vi "Result_Test.vi"(8 "error in (no error)":errorcluster caption="entrée d'erreur (pas d'erreur)", 11 "Nodon_Get_Power IN":refnum<class "Nodon_Get_Power.lvclass">) -> (0 "error out":errorcluster caption="sortie d'erreur", 3 "Nodon_Get_Power OUT":refnum<class "Nodon_Get_Power.lvclass">)   [LabVIEW 2020, in "Library Test.lvlib" / "Nodon_Get_Power.lvclass"]
uses:
  Nodon_Get_Power.lvclass
  C:/Users/ngarcin/OneDrive - Altyor/Standard TB/Suite TB45/Class/Test/Test (Default)/Test (Default).lvclass
  Commun VI/TypeDef/Variable Printable.ctl
  JSON API/JSON Value/Set from JSON string.vi
  JSON API/JSON Value/JSON Value.lvclass
  Nodon_Send_Command_UART.lvclass
  JSON API/Variant JSON/Variant JSON.lvlib
  JSON API/Get Polymorphic/JSON GetSet.lvlib
  Commun VI/Library Commun.lvlib
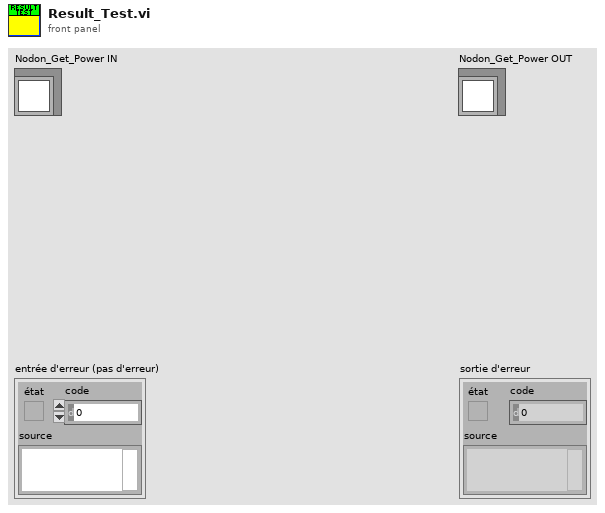
[diagram p1: front panel]
types:
  T1 = typedef "Variable Printable.ctl" = string
  T2 = enum16{"Get Variable", "Get All Variables", "Set Variable", "Delete Variable", "Delete All Variable"}
  T3 = cluster{"Commande Type":string, "Command ID":string, "Data":string, "Error":string}
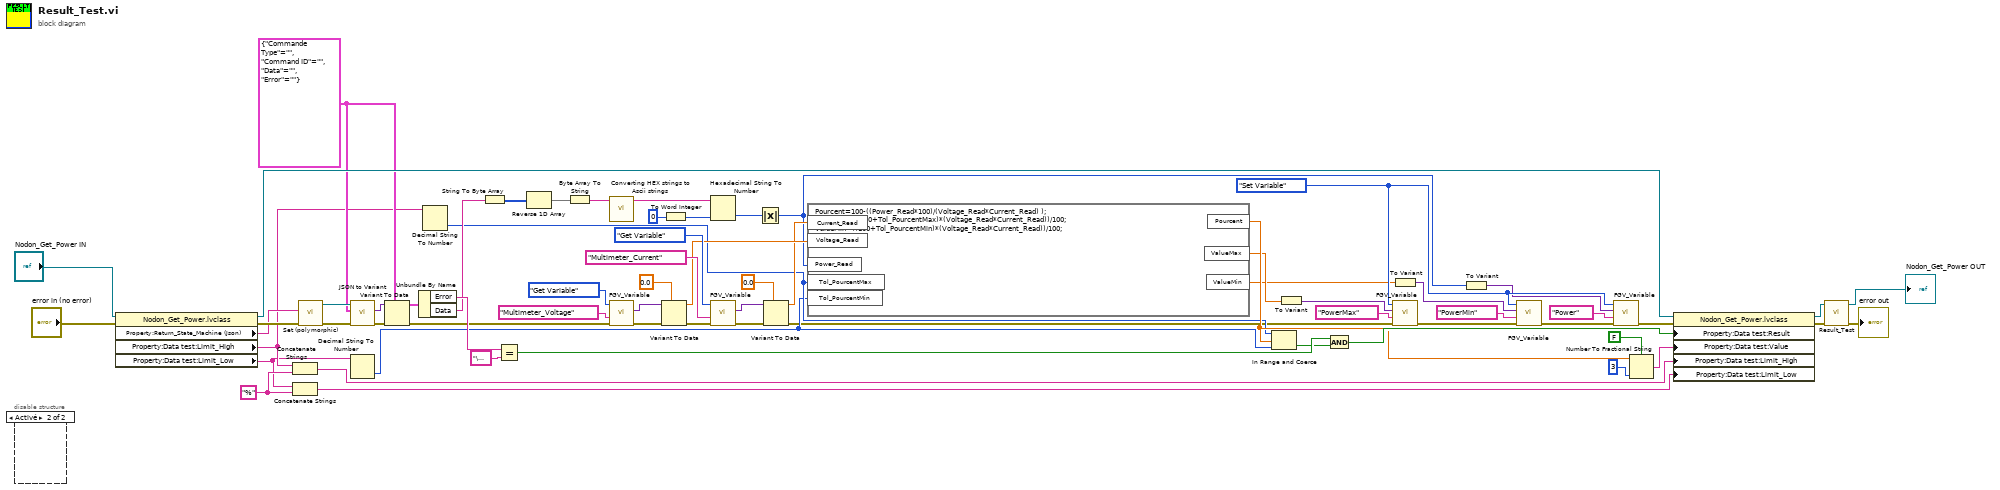
[diagram p0: block diagram]
diagram:
  w9 = T2."Set Variable" ("Function")
  w41 = "%" ("chaîne")
  w54 = T3 {"Commande Type"="", "Command ID"="", "Data"="", "Error"=""}
  n1 = disable-structure shown="Activé" {
    frame Disabled {
    }
    frame Enabled {
    }
  }
  n2 = property class="Nodon_Get_Power.lvclass"(reference="Nodon_Get_Power IN", error in="error in (no error)") -> (reference out=w65:refnum<class "Nodon_Get_Power.lvclass">, error out=w60:errorcluster, "Property:Return_State_Machine (Json)"=w59:string, "Property:Data test:Limit_High"=w24:string, "Property:Data test:Limit_Low"=w23:string)
  n3 = Concatenate Strings(w24, w41) -> (w40:string)
  n4 = Concatenate Strings(w23, w41) -> (w39:string)
  n5 = call-poly "Set (polymorphic).vi"("error in (no error)"=w60, "JSON stream"=w59) -> ("error out"=w62:errorcluster, "JSON Value out"=w64:refnum<class "JSON Value.lvclass">)  [unwired: 7 in, 1 out]
  n6 = call "JSON to Variant.vi"("error in (no error)"=w62, "Variant (Data Type)"=w54, "JSON Value"=w64) -> ("error out"=w63:errorcluster, "Variant out"=w61:variant)  [unwired: 7 in]
  n7 = Decimal String To Number(string=w23) -> (number=w17:i32)  [unwired: 2 in, 1 out]
  n8 = Variant To Data(error in=w63, type=w54, Variant=w61) -> (data=w58:T3, error out=w27:errorcluster)
  n9 = Unbundle By Name(w58) -> ("Error"=w57:string, "Data"=w42:string)
  n10 = Decimal String To Number(string=w24) -> (number=w18:i32)  [unwired: 2 in, 1 out]
  n11 = String To Byte Array(string=w42) -> (unsigned byte array=w44:u8[])
  n12 = Equal?(x=w57, y="\u0000") -> (x = y?=w55:bool)
  n13 = Reverse 1D Array(array=w44) -> (reversed array=w45:u8[])
  n14 = Byte Array To String(unsigned byte array=w45) -> (string=w48:string)
  n15 = call "Converting HEX strings to Ascii strings.vi"("chaîne IN"=w48) -> ("Chaîne OUT"=w49:string)  [unwired: 9 in, 1 out]
  n16 = call "FGV_Variable.vi"("error in (no error)"=w27, "Variable"=T1 "Multimeter_Voltage", "Function"=T2."Get Variable") -> ("error out"=w36:errorcluster, "Data Out"=w35:variant)  [unwired: 6 in, 1 out]
  n17 = Variant To Data(error in=w36, type=0.0, Variant=w35) -> (data=w26:dbl, error out=w28:errorcluster)
  n18 = To Word Integer(number=i16 0 ("nombre")) -> (16bit integer=w47:i16)
  n19 = Hexadecimal String To Number(string=w49, default (0uL)=w47) -> (number=w46:i16)  [unwired: 1 in, 1 out]
  n20 = call "FGV_Variable.vi"("error in (no error)"=w28, "Variable"=T1 "Multimeter_Current", "Function"=T2."Get Variable") -> ("error out"=w31:errorcluster, "Data Out"=w30:variant)  [unwired: 6 in, 1 out]
  n21 = Absolute Value(x=w46) -> (abs(x)=w3:i16)
  n22 = Variant To Data(error in=w31, type=0.0, Variant=w30) -> (data=w25:dbl, error out=w16:errorcluster)
  n23 = formula code="Pourcent=100-((Power_Read*100)/(Voltage_Read*Current_Read) );\nValueMax=((100+Tol_PourcentMax)*(Voltage_Read*Current_Read))/100;\nValueMin=((100+Tol_PourcentMin)*(Voltage_Read*Current_Read))/100;"("Voltage_Read"=w26, "Current_Read"=w25, "Power_Read"=w3, "Tol_PourcentMax"=w18, "Tol_PourcentMin"=w17) -> ("Pourcent"=w19:dbl, "ValueMax"=w14:dbl, "ValueMin"=w8:dbl)
  n24 = In Range and Coerce(upper limit=w18, x=w19, lower limit=w17) -> (In Range?=w21:bool)  [unwired: 1 out]
  n25 = To Variant(anything=w14) -> (Variant=w13:variant)
  n26 = Compound Arithmetic op=AND ("Opérateur arithmétique")(w55, w21) -> (w22:bool)
  n27 = call "FGV_Variable.vi"("error in (no error)"=w16, "Variable"=T1 "PowerMax", "Data In"=w13, "Function"=w9) -> ("error out"=w12:errorcluster)  [unwired: 5 in, 2 out]
  n28 = To Variant(anything=w8) -> (Variant=w6:variant)
  n29 = To Variant(anything=w3) -> (Variant=w4:variant)
  n30 = call "FGV_Variable.vi"("error in (no error)"=w12, "Variable"=T1 "PowerMin", "Data In"=w6, "Function"=w9) -> ("error out"=w11:errorcluster)  [unwired: 5 in, 2 out]
  n31 = call "FGV_Variable.vi"("error in (no error)"=w11, "Variable"=T1 "Power", "Data In"=w4, "Function"=w9) -> ("error out"=w10:errorcluster)  [unwired: 5 in, 2 out]
  n32 = Number To Fractional String(use system decimal point (T)=FALSE ("utiliser le séparateur décimal du système (V)"), number=w19, precision (6)=i16 3 ("précision (6)")) -> (F-format string=w20:string)  [unwired: 1 in]
  n33 = property class="Nodon_Get_Power.lvclass"(reference=w65, error in=w10, "Property:Data test:Result"=w22, "Property:Data test:Value"=w20, "Property:Data test:Limit_High"=w40, "Property:Data test:Limit_Low"=w39) -> (reference out=w51:refnum<class "Nodon_Get_Power.lvclass">, error out=w50:errorcluster)
  n34 = call-parent "Result_Test.vi"("error in (no error)"=w50, "Get_Voltage en entrée"=w51) -> ("error out"=→"error out":errorcluster, "Get_Voltage en sortie"=→"Nodon_Get_Power OUT":refnum<class "Nodon_Get_Power.lvclass">)  [unwired: 8 in]
